vi "FindChildActorAttribs.vi"(10 "Alias":string, 11 "Actor":T1) -> (2 "ChildActorAttribs":T2, 3 "Found":bool)   [LabVIEW 2020, in "jettl.lvlib"]
uses:
  jettl.lvlib
  Metadata/Metadata.lvclass
  Msg/Msg.lvclass
  MsgNames.ctl
  Msg.ctl
  ActorAttribs.ctl
  PostSetup.ctl
  PreSetup.ctl
  Lifecycle.ctl
  Origin.ctl
  MsgAttribs.ctl
  MsgExecuteType.ctl
  ChildActors.ctl
  Actor.ctl
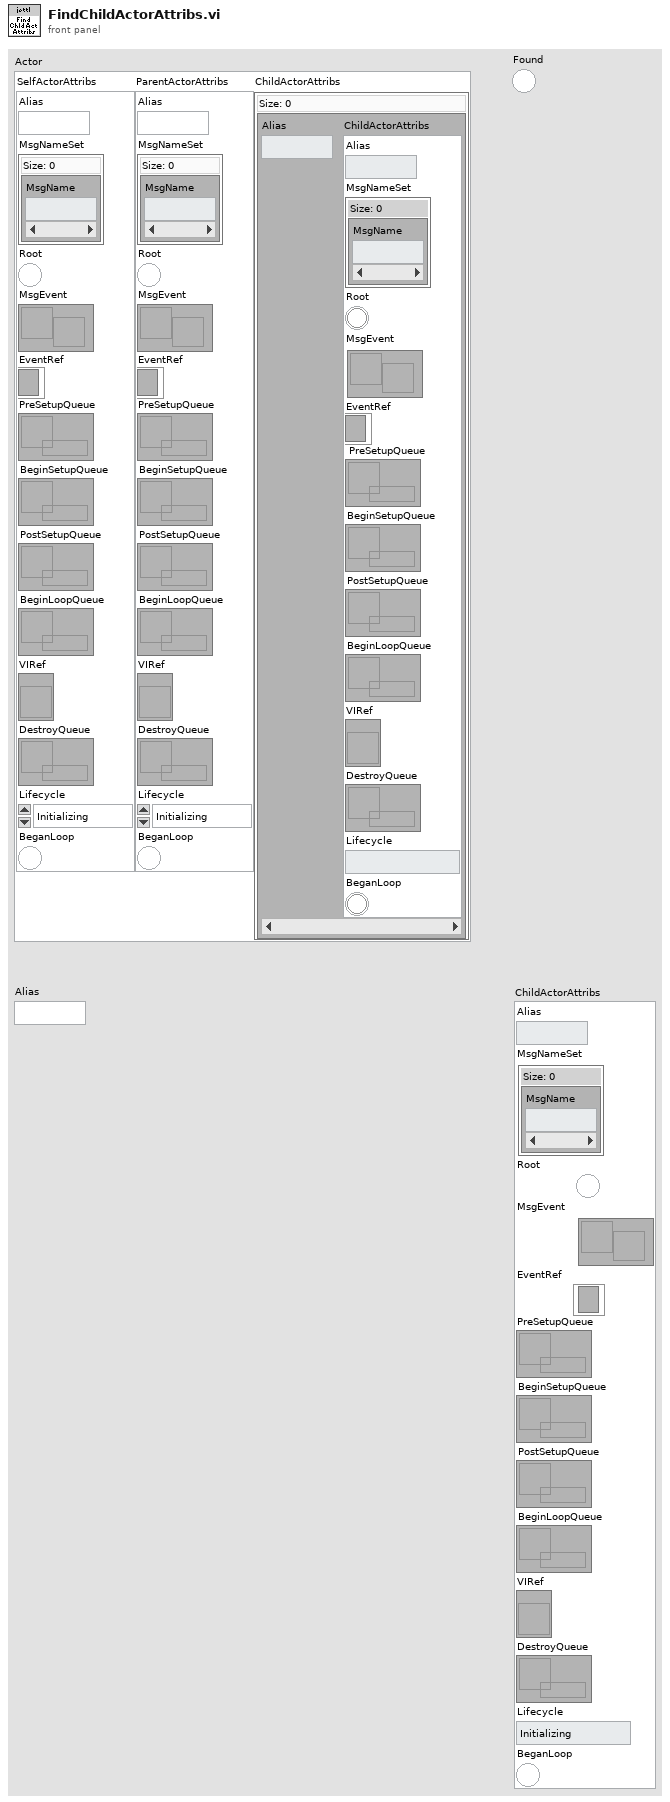
[diagram p1: front panel]
types:
  T1 = typedef "jettl.lvlib/Actor.ctl" = cluster{"SelfActorAttribs":T2, "ParentActorAttribs":T2, "ChildActorAttribs":T5}
  T2 = typedef "jettl.lvlib/ActorAttribs.ctl" = cluster{"Alias":string, "MsgNameSet":T3, "Root":bool, "MsgEvent":refnum<user-event>, "EventRef":refnum<event-registration>, "PreSetupQueue":refnum<queue>, "BeginSetupQueue":refnum<queue>, "PostSetupQueue":refnum<queue>, "BeginLoopQueue":refnum<queue>, "VIRef":refnum<vi>, "DestroyQueue":refnum<queue>, "Lifecycle":T4, "BeganLoop":bool}
  T3 = typedef "jettl.lvlib/MsgNames.ctl" = set{string}
  T4 = typedef "jettl.lvlib/Lifecycle.ctl" = enum16{"Initializing", "SettingUp", "Starting", "Running", "Stopping", "TearingDown", "Terminated"}
  T5 = typedef "jettl.lvlib/ChildActors.ctl" = map{string, T2}
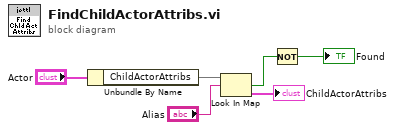
[diagram p0: block diagram]
diagram:
  n1 = Unbundle By Name("Actor") -> ("ChildActorAttribs"=w2:T5)
  n2 = Look In Map(map=w2, key="Alias") -> (key not found?=w4:bool, value=→"ChildActorAttribs":T2)  [unwired: 1 in]
  n3 = Not(x=w4) -> (.not. x?=→"Found":bool)
